vi "Example Three Stage.vi"() -> ()   [LabVIEW 2019]
uses:
  Class/Controller/Controller.lvclass
  <vilib>/Platform/TimedLoop/XDataNode/timing_clust.ctl
  <vilib>/Platform/TimedLoop/XDataNode/nitl_modes.ctl
  <vilib>/Platform/TimedLoop/XDataNode/wakeup.ctl
  <vilib>/platform/TimedLoop/XDataNode/XDataNode.xnode
  <vilib>/Platform/TimedLoop/XDataNode/XDNodeRunTimeDep.lvlib
panel:
  in  "Tab Control 3":enum32{"Motion", "Settings"}(tab)
  in  "Zero Output 3":bool
  in  "Go to Home 3":bool
  in  "Scan Right 3":bool
  in  "Scan Left 3":bool
  in  "Continue 3":bool
  in  "Stop 3":bool
  in  "Make Step Right 3":bool
  in  "Step Size \n[selected units] 3":dbl=1.0 format="%#.2f"
  in  "Make Step Left 3":bool
  in  "Desired Speed \n[1µm/s or 0,01deg /s] 3":dbl=10000.0 format="%#.2f"
  in  "Desired Position \n[selected units] 3":dbl format="%#.2f"
  in  "Find Index 3":bool
  in  "Reset 3":bool
  out "Desired Position\n[selected units] 3":dbl
  out "Encoder position \n[selected units] 3":dbl
  out "Waveform Chart 3":dbl(graph)=-0.078
  out "Status Info 3":T1
  out "StatusBits 3":T2
  in  "Working Units 3":string(combo)="1000000"
  in  "Axis Resolution 3":string(combo)="312,5"
  in  "Axis Letter 3":string="Z"
  in  "Tab Control 2":enum32{"Motion", "Settings"}(tab)
  in  "Zero Output 2":bool
  in  "Go to Home 2":bool
  in  "Scan Right 2":bool
  in  "Scan Left 2":bool
  in  "Continue 2":bool
  in  "Stop 2":bool
  in  "Make Step Right 2":bool
  in  "Step Size \n[selected units] 2":dbl=1.0 format="%#.2f"
  in  "Make Step Left 2":bool
  in  "Desired Speed \n[1µm/s or 0,01deg /s] 2":dbl=10000.0 format="%#.2f"
  in  "Desired Position \n[selected units] 2":dbl format="%#.2f"
  in  "Find Index 2":bool
  in  "Reset 2":bool
  out "Desired Position\n[selected units] 2":dbl
  out "Encoder position \n[selected units] 2":dbl
  out "Waveform Chart 2":dbl(graph)=-0.078
  out "Status Info 2":T1
  out "StatusBits 2":T2
  out "Desired Position\n[selected units]":dbl
  out "Encoder position \n[selected units]":dbl
  in  "Tab Control":enum32{"Motion", "Settings"}(tab)
  in  "Zero Output":bool
  in  "Go to Home":bool
  in  "Scan Right":bool
  in  "Scan Left":bool
  in  "Continue":bool
  in  "Stop":bool
  in  "Make Step Right":bool
  in  "Step Size \n[selected units]":dbl=1.0 format="%#.2f"
  in  "Make Step Left":bool
  in  "Desired Speed \n[1µm/s or 0,01deg /s]":dbl=10000.0 format="%#.2f"
  in  "Desired Position \n[selected units]":dbl format="%#.2f"
  in  "Find Index":bool
  in  "Reset":bool
  out "error out":errorcluster
  in  "Working Units 2":string(combo)="1000000"
  in  "Working Units":string(combo)="1000000"
  out "StatusBits":T2
  out "Status Info":T1
  in  "Axis Resolution 2":string(combo)="312,5"
  in  "Axis Letter 2":string="Y"
  in  "Axis Resolution":string(combo)="312,5"
  in  "Axis Letter":string="X"
  in  "Baudrate":dbl=9600.0
  in  "COM Port":refnum<visa-resource-name>
  in  "Controller.lvclass":refnum<class "Controller.lvclass">
  out "Waveform Chart":dbl(graph)=-0.078
  in  "STOP PROGRAM":bool
  # "Visualization"
  # "Extra information"
  # "READ ME FIRST"
  # "Configuration"
  # "Stage 1"
  # "Driver 1"
  # "Stage 1"
  # "How to run:"
  # "BEFORE RUNNING:"
  # "1, Select COM Port"
  # "2. Select baudrate"
  # "3. For each axis:"
  # "3.1 Specify correct axis name (1 letter)"
  # "3.2 Specify correct resolution"
  # "4. Run VI"
  # "WHEN RUNNING, YOU HAVE TO FIRST PUSH \"FIND INDEX\" FOR EACH STAGE.\nThe stages will start moving and find its position. After that you can control the stages"
  # "Stage 2"
  # "NOTES: Do this only the first time"
  # "1. Replace the settings_default.txt file with\nthe file we provided on a USB stick."
  # "2.    Make sure there are no comments in the\nsettings_default.txt file. ONLY lines like: \"X:DPOS=100\" so NO \"%\" in front or at the end of the line."
  # "Position Information"
  # "Stage 3"
  # "3.  In your settings_default.txt file:\nEvery line that contains SSPD or MSPD: multiply that value with:\n - 1000 for a lineair stage \n - 100 for a rotating stage"
  # "STOP BUTTON"
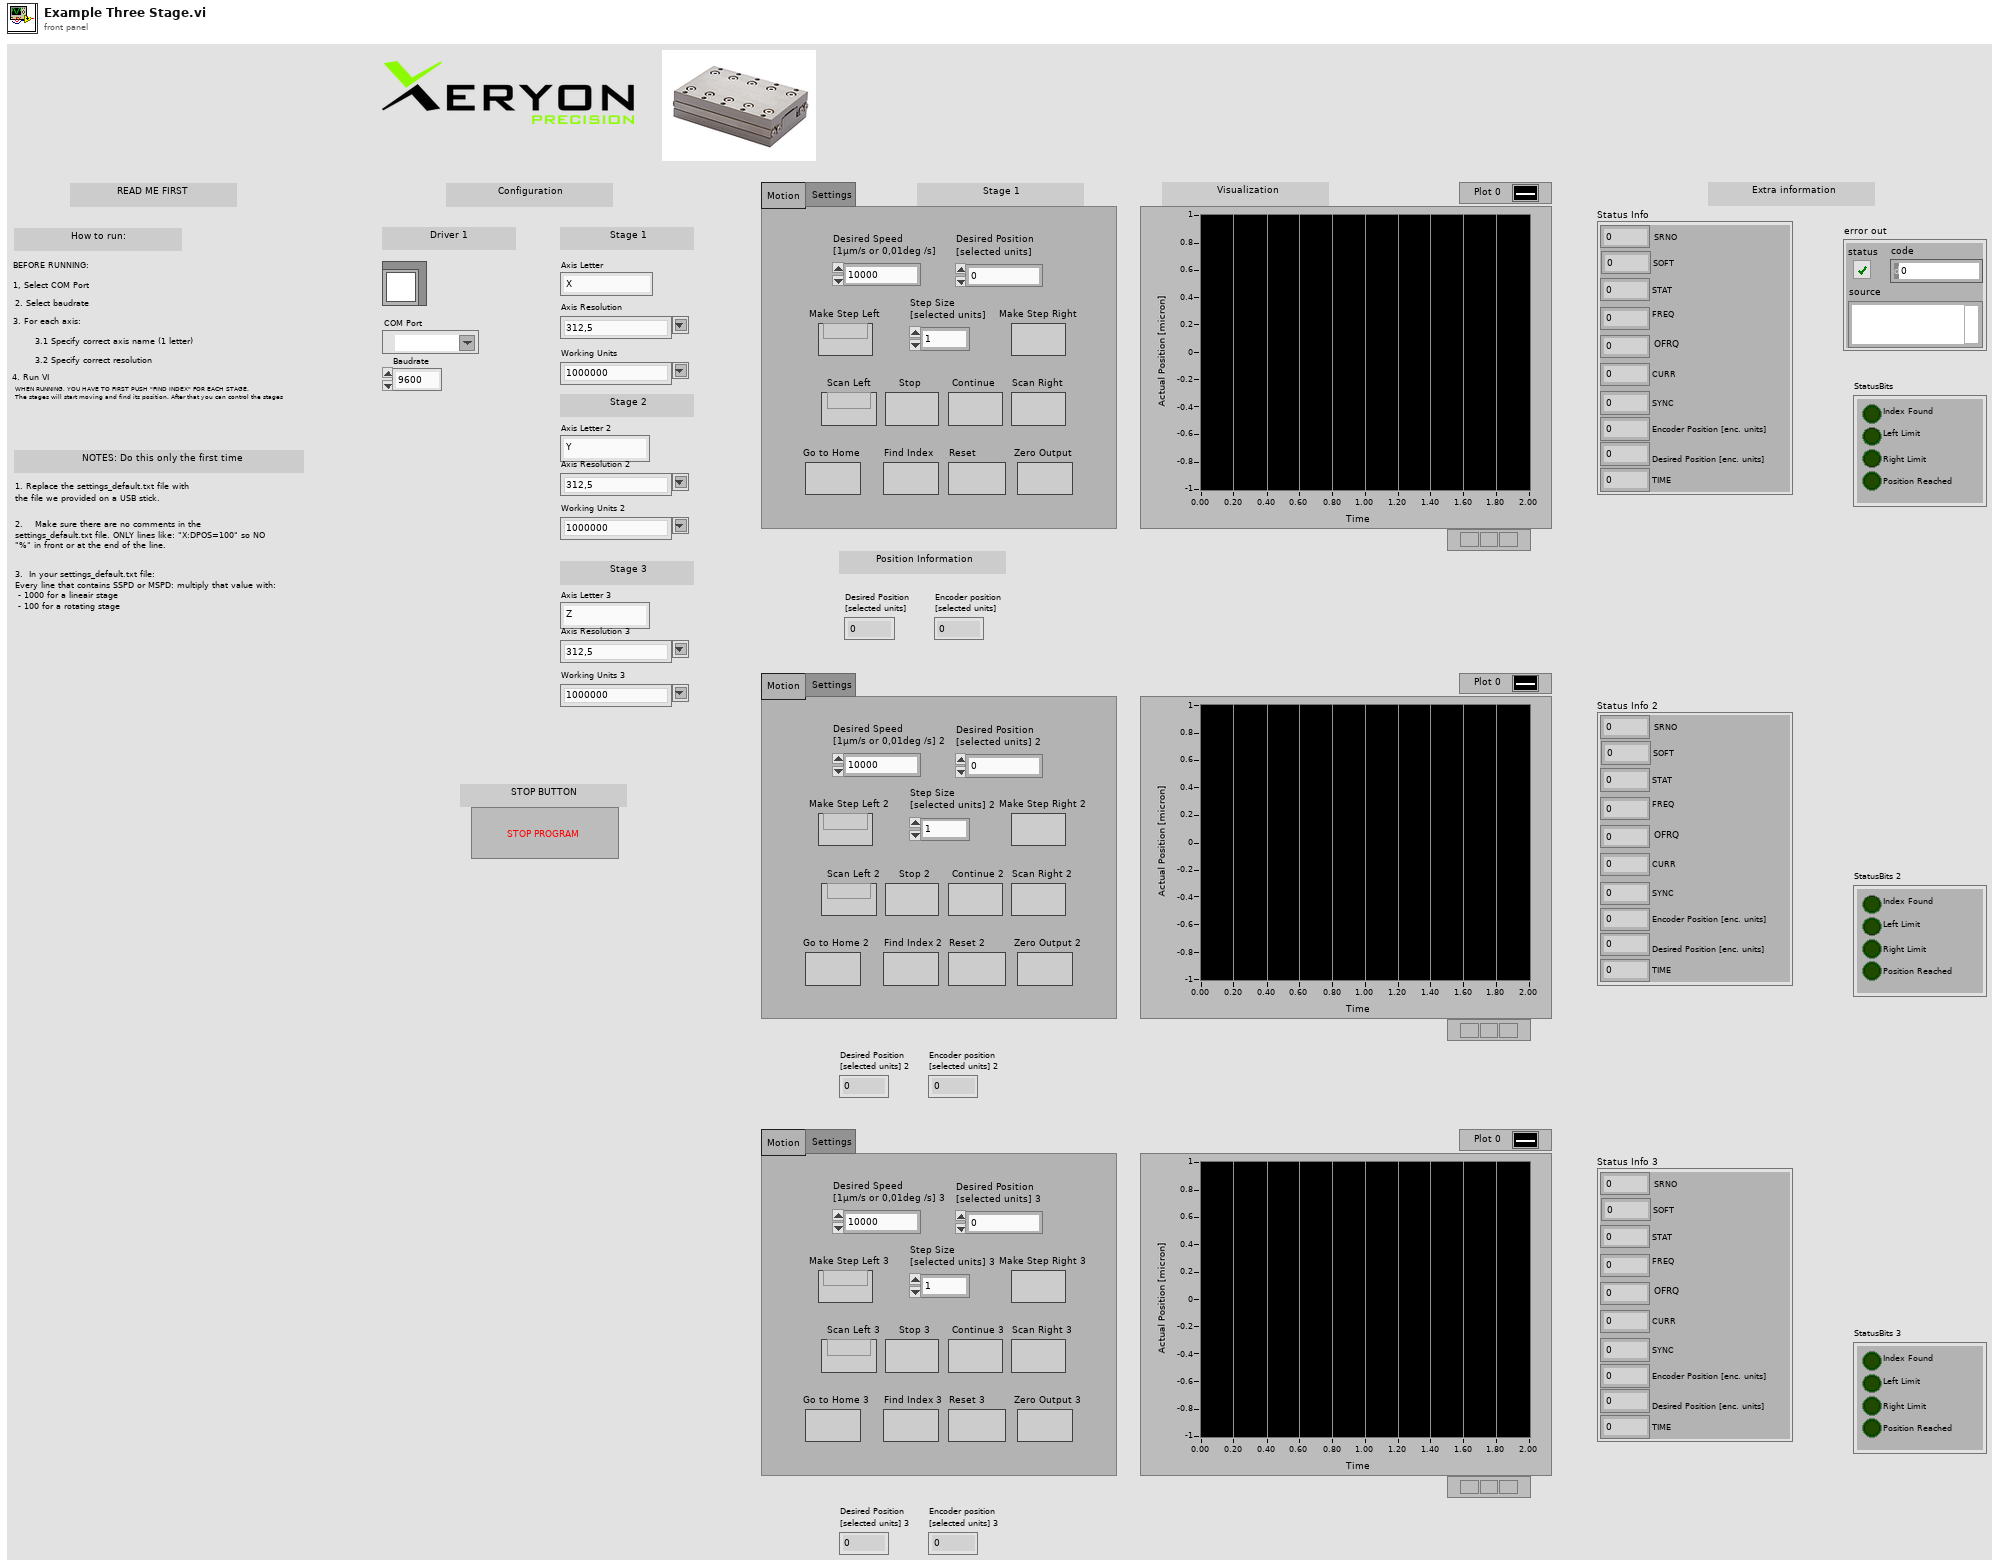
[diagram p1: front panel]
types:
  T1 = cluster{"SRNO":dbl, "SOFT":dbl, "STAT":dbl, "FREQ":dbl, "OFRQ":dbl, "CURR":dbl, "SYNC":dbl, "Encoder Position [enc. units]":dbl, "Desired Position [enc. units]":dbl, "TIME":dbl}
  T2 = cluster{"Index Found":bool, "Left Limit":bool, "Right Limit":bool, "Position Reached":bool}
  T3 = typedef "XDNodeRunTimeDep.lvlib/timing_clust.ctl" = cluster{"Expected End [f-1]":u64, "Actual End [f-1]":u64, "Finished Late? [f-1]":bool, "Expected End [i-1]":u64, "Actual End [i-1]":u64, "Finished Late? [i-1]":bool, "Expected Start [i]":u64, "Actual Start [i]":u64, "Expected Start [f]":u64, "Actual Start [f]":u64, "Source Name":string, "Structure Name":string, "Period":i64, "Deadline":i64, "Offset":i64, "Start":i64, "Priority":i32, "Timeout":i32, "Mode":T4, "Wakeup Reason":T5, "Error":errorcluster, "Source Type":string, "Secondary Source Type":string, "Global End Time":u64, "Global Start Time":u64, "Frame Duration":u64, "Iteration Duration":u64, "Assigned CPU":i32, "I/O Scan Engine Mode":u32}
  T4 = typedef "XDNodeRunTimeDep.lvlib/nitl_modes.ctl" = enum32{"No Change", "Process missed periods, maintain original phase", "Discard missed periods, maintain original phase", "Process missed periods, ignore original phase", "Discard missed periods, ignore original phase"}
  T5 = typedef "XDNodeRunTimeDep.lvlib/wakeup.ctl" = enum32{"Normal", "Aborted", "Asynchronous wakeup", "Timing source error", "Timed loop error", "Timeout"}
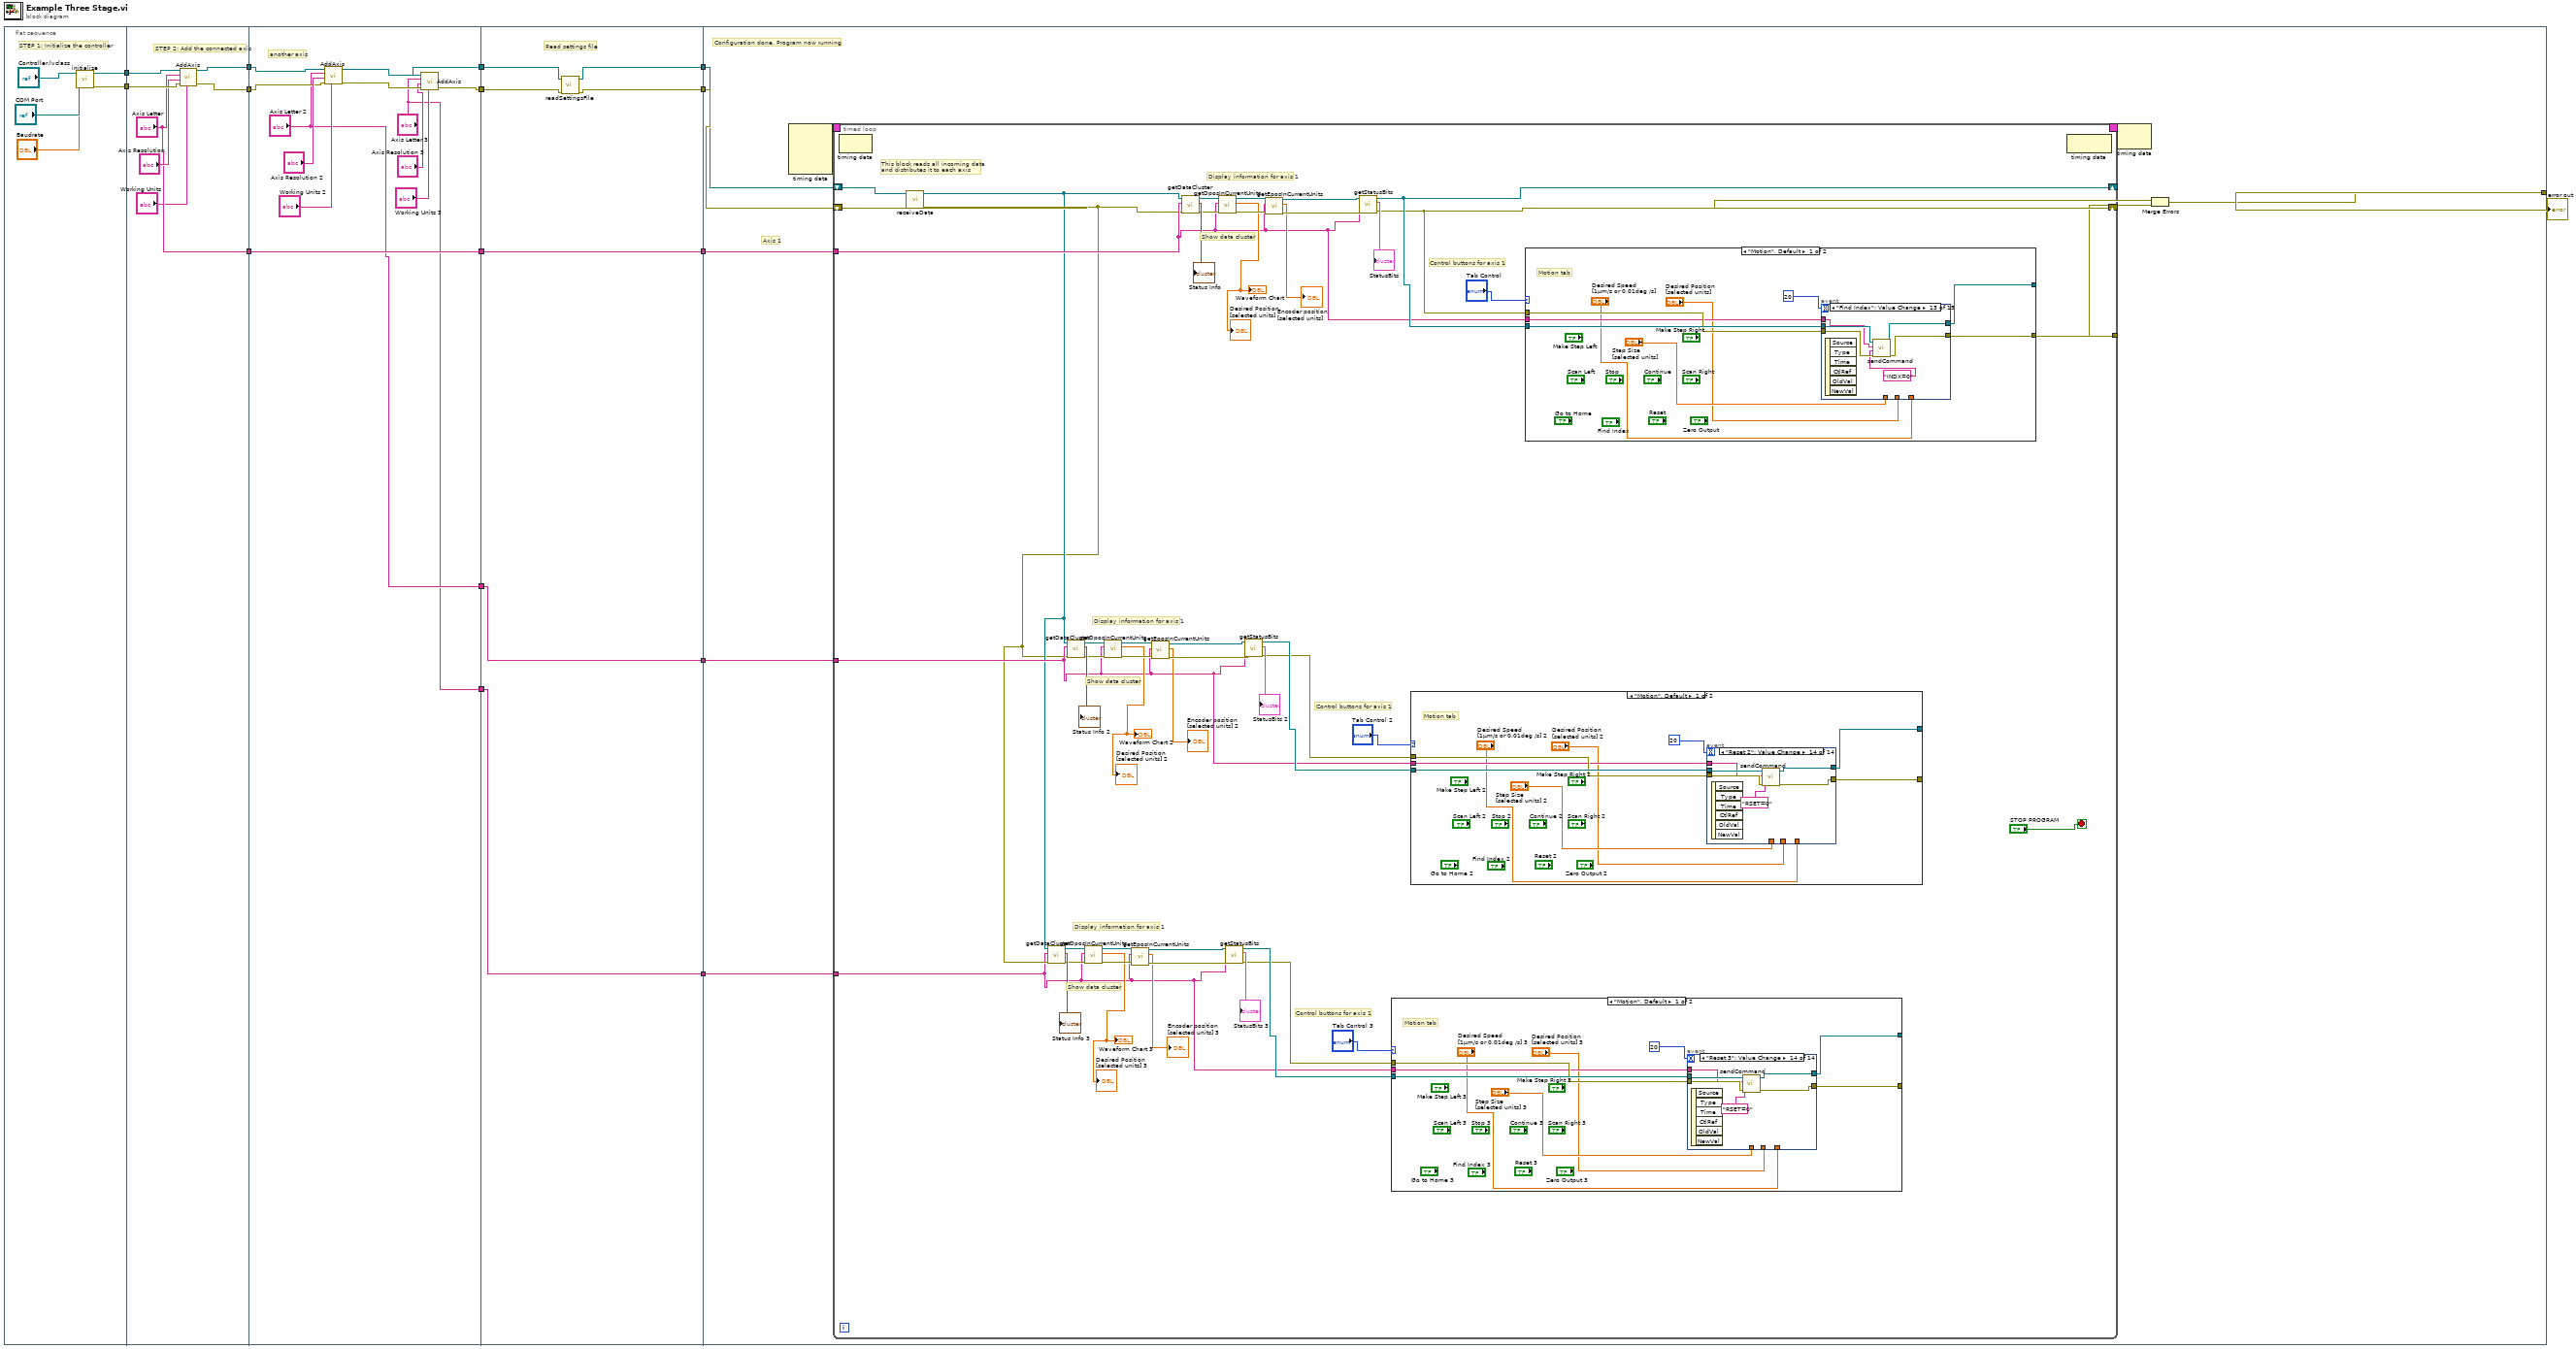
[diagram p0: block diagram]
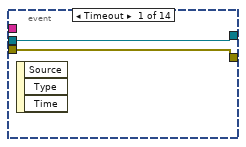
[diagram p2: hidden frame]
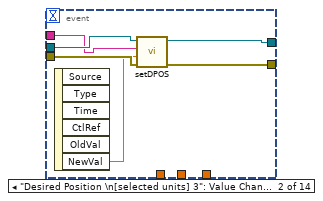
[diagram p3: hidden frame]
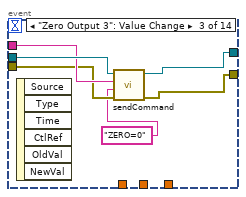
[diagram p4: hidden frame]
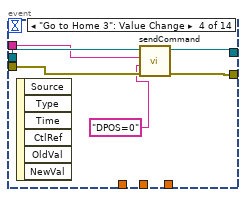
[diagram p5: hidden frame]
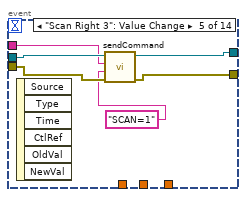
[diagram p6: hidden frame]
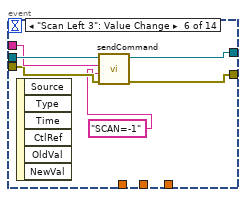
[diagram p7: hidden frame]
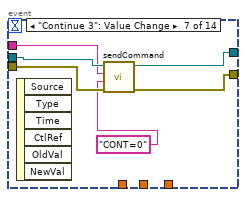
[diagram p8: hidden frame]
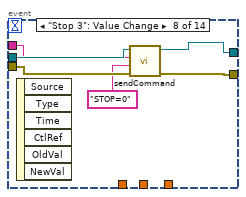
[diagram p9: hidden frame]
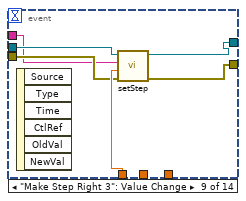
[diagram p10: hidden frame]
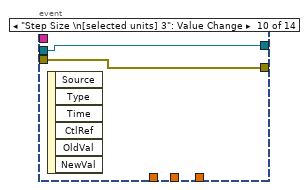
[diagram p11: hidden frame]
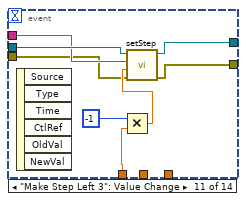
[diagram p12: hidden frame]
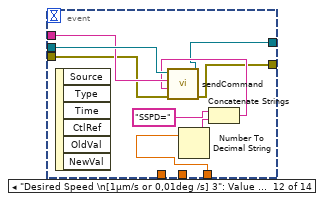
[diagram p13: hidden frame]
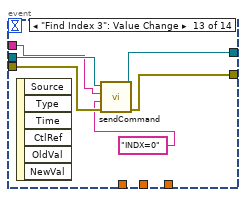
[diagram p14: hidden frame]
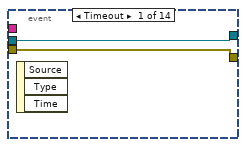
[diagram p16: hidden frame]
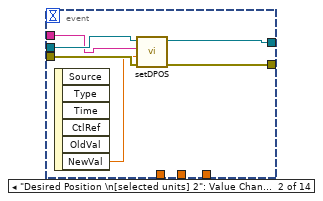
[diagram p17: hidden frame]
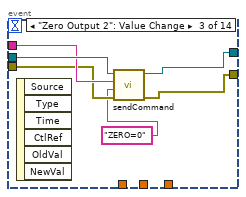
[diagram p18: hidden frame]
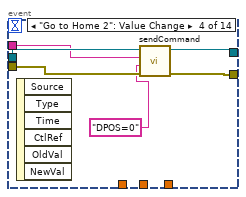
[diagram p19: hidden frame]
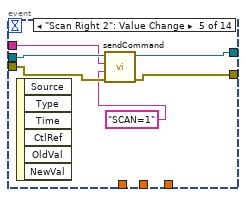
[diagram p20: hidden frame]
diagram:
  n1 = flat-sequence {
    tunnel: [w18] -> w16
    tunnel: [w17] -> w15
    tunnel: w16 -> [w28]
    tunnel: w15 -> [w27]
    tunnel: [w25] -> w14
    tunnel: [w24] -> w13
    tunnel: ["Axis Letter"] -> w12
    tunnel: w14 -> [w39]
    tunnel: w13 -> [w38]
    tunnel: [w41] -> w10
    tunnel: w12 -> [w41]
    tunnel: [w34] -> w8
    tunnel: [w32] -> w6
    tunnel: ["Axis Letter 2"] -> w4
    tunnel: ["Axis Letter 3"] -> w1
    tunnel: w10 -> [w48]
    tunnel: [w48] -> w9
    tunnel: w8 -> [w47]
    tunnel: [w45] -> w7
    tunnel: w6 -> [w46]
    tunnel: [w44] -> w5
    tunnel: w4 -> [w43]
    tunnel: [w43] -> w3
    tunnel: [w42] -> w2
    tunnel: w1 -> [w42]
    tunnel: w9 -> [w51]
    tunnel: w7 -> [w57]
    tunnel: w5 -> [w58]
    tunnel: [w53] -> w11
    tunnel: w3 -> [w50]
    tunnel: w2 -> [w49]
    frame #0 {
      # "STEP 1: Initialize the controller"
      n2 = call-dynamic "initialize.vi"("Baudrate"="Baudrate", "COM Port"="COM Port", "Controller in"="Controller.lvclass") -> ("error out"=w17:errorcluster, "Controller out"=w18:refnum<class "Controller.lvclass">)  [unwired: 7 in]
    }
    frame #1 {
      # "STEP 2: Add the connected axis"
      n3 = call-dynamic "AddAxis.vi"("Units"="Working Units", "error in (no error)"=w27, "Encoder Resolution"="Axis Resolution", "Axis Letter"="Axis Letter", "Controller in"=w28) -> ("error out"=w24:errorcluster, "Controller out"=w25:refnum<class "Controller.lvclass">)  [unwired: 5 in]
    }
    frame #2 {
      # "another axis"
      n4 = call-dynamic "AddAxis.vi"("Units"="Working Units 2", "error in (no error)"=w38, "Encoder Resolution"="Axis Resolution 2", "Axis Letter"="Axis Letter 2", "Controller in"=w39) -> ("error out"=w33:errorcluster, "Controller out"=w35:refnum<class "Controller.lvclass">)  [unwired: 5 in]
      n5 = call-dynamic "AddAxis.vi"("Units"="Working Units 3", "error in (no error)"=w33, "Encoder Resolution"="Axis Resolution 3", "Axis Letter"="Axis Letter 3", "Controller in"=w35) -> ("error out"=w32:errorcluster, "Controller out"=w34:refnum<class "Controller.lvclass">)  [unwired: 5 in]
    }
    frame #3 {
      # "Read settings file"
      n6 = call-dynamic "readSettingsFile.vi"("error in (no error)"=w46, "Controller in"=w47) -> ("error out"=w44:errorcluster, "Controller out"=w45:refnum<class "Controller.lvclass">)  [unwired: 8 in]
    }
    frame #4 {
      # "Axis 1"
      # "Configuration done. Program now running"
      n7 = node-c288() -> (w56:T3)  [unwired: 4 in]
      n8 = timed-loop {
        shift-right: [w92] -> _
        shift-left: w57 -> [w106]
        tunnel: w51 -> [w90]
        shift-right: [w91] -> w54
        shift-left: w58 -> [w95]
        timing: w56 -> [_]
        timing-out: [_] -> w55
        tunnel: [w89] -> w52
        tunnel: w50 -> [w75]
        tunnel: w49 -> [w59]
        stop <- "STOP PROGRAM" stop-if-true
        # "Control buttons for axis 1"
        # "Display information for axis 1"
        # "Show data cluster"
        # "Control buttons for axis 1"
        # "Display information for axis 1"
        # "Show data cluster"
        # "Control buttons for axis 1"
        # "Display information for axis 1"
        # "Show data cluster"
        # "This block reads all incoming data\nand distributes it to each axis"
        n9 = node-c288() -> ()  [unwired: 1 in, 1 out]
        n10 = call-dynamic "receiveData.vi"("error in (no error)"=w95, "Controller in"=w106) -> ("error out"=w60:errorcluster, "Controller out"=w61:refnum<class "Controller.lvclass">)  [unwired: 8 in]
        n11 = call-dynamic "getDataCluster.vi"("error in (no error)"=w60, "Axis Letter"=w59, "Controller in"=w61) -> ("error out"=w69:errorcluster, "Information"=→"Status Info 3":T1, "Controller out"=w72:refnum<class "Controller.lvclass">)  [unwired: 6 in]
        n12 = call-dynamic "getDataCluster.vi"("error in (no error)"=w60, "Axis Letter"=w75, "Controller in"=w61) -> ("error out"=w83:errorcluster, "Information"=→"Status Info 2":T1, "Controller out"=w86:refnum<class "Controller.lvclass">)  [unwired: 6 in]
        n13 = call-dynamic "getDposInCurrentUnits.vi"("error in (no error)"=w69, "Axis Letter"=w59, "Controller in"=w72) -> ("error out"=w68:errorcluster, "DPOS In Current Units"=→"Waveform Chart 3" →"Desired Position\n[selected units] 3":dbl, "Controller out"=w71:refnum<class "Controller.lvclass">)  [unwired: 6 in]
        n14 = call-dynamic "getDposInCurrentUnits.vi"("error in (no error)"=w83, "Axis Letter"=w75, "Controller in"=w86) -> ("error out"=w82:errorcluster, "DPOS In Current Units"=→"Waveform Chart 2" →"Desired Position\n[selected units] 2":dbl, "Controller out"=w85:refnum<class "Controller.lvclass">)  [unwired: 6 in]
        n15 = call-dynamic "getEposInCurrentUnits.vi"("error in (no error)"=w68, "Axis Letter"=w59, "Controller in"=w71) -> ("error out"=w67:errorcluster, "EPOS In Current Units"=→"Encoder position \n[selected units] 3":dbl, "Controller out"=w70:refnum<class "Controller.lvclass">)  [unwired: 6 in]
        n16 = call-dynamic "getEposInCurrentUnits.vi"("error in (no error)"=w82, "Axis Letter"=w75, "Controller in"=w85) -> ("error out"=w81:errorcluster, "EPOS In Current Units"=→"Encoder position \n[selected units] 2":dbl, "Controller out"=w84:refnum<class "Controller.lvclass">)  [unwired: 6 in]
        n17 = call-dynamic "getDataCluster.vi"("error in (no error)"=w60, "Axis Letter"=w90, "Controller in"=w61) -> ("error out"=w100:errorcluster, "Information"=→"Status Info":T1, "Controller out"=w103:refnum<class "Controller.lvclass">)  [unwired: 6 in]
        n18 = call-dynamic "getDposInCurrentUnits.vi"("error in (no error)"=w100, "Axis Letter"=w90, "Controller in"=w103) -> ("error out"=w99:errorcluster, "DPOS In Current Units"=→"Waveform Chart" →"Desired Position\n[selected units]":dbl, "Controller out"=w102:refnum<class "Controller.lvclass">)  [unwired: 6 in]
        n19 = call-dynamic "getStatusBits.vi"("error in (no error)"=w67, "Axis Letter"=w59, "Controller in"=w70) -> ("error out"=w62:errorcluster, "StatusBits"=→"StatusBits 3":T2, "Controller out"=w63:refnum<class "Controller.lvclass">)  [unwired: 6 in]
        n20 = call-dynamic "getStatusBits.vi"("error in (no error)"=w81, "Axis Letter"=w75, "Controller in"=w84) -> ("error out"=w76:errorcluster, "StatusBits"=→"StatusBits 2":T2, "Controller out"=w77:refnum<class "Controller.lvclass">)  [unwired: 6 in]
        n21 = call-dynamic "getEposInCurrentUnits.vi"("error in (no error)"=w99, "Axis Letter"=w90, "Controller in"=w102) -> ("error out"=w98:errorcluster, "EPOS In Current Units"=→"Encoder position \n[selected units]":dbl, "Controller out"=w101:refnum<class "Controller.lvclass">)  [unwired: 6 in]
        n22 = call-dynamic "getStatusBits.vi"("error in (no error)"=w98, "Axis Letter"=w90, "Controller in"=w101) -> ("error out"=w91:errorcluster, "StatusBits"=→"StatusBits":T2, "Controller out"=w92:refnum<class "Controller.lvclass">)  [unwired: 6 in]
        n23 = case shown="\"Motion\", Default" "Tab Control 3" {
          tunnel: w63 -> [w115 w197]
          tunnel: w62 -> [w114 w198]
          tunnel: [w113 w197] -> _
          tunnel: [w112 w198] -> _
          tunnel: w59 -> [w110 _]
          frame "Motion", Default {
            # "Motion tab"
            n24 = event shown="[13] \"Reset 3\": Value Change" {
              selector: _ -> [_ _ _ _ _ _ _ _ _ _ _ _ _ _]
              dyn-events: _ -> [_ _ _ _ _ _ _ _ _ _ _ _ _ _]
              timeout: 20 -> [_ _ _ _ _ _ _ _ _ _ _ _ _ _]
              tunnel: w115 -> [w117 w123 w129 w135 w141 w147 w153 w159 w163 w167 w173 w184 w190 w196]
              tunnel: w114 -> [w116 w122 w127 w133 w139 w145 w151 w157 w164 w166 w170 w182 w188 w195]
              tunnel: [w117 w120 w125 w130 w137 w143 w149 w155 w161 w167 w168 w176 w186 w192] -> w113
              tunnel: [w116 w121 w126 w132 w138 w144 w150 w156 w160 w166 w169 w177 w187 w191] -> w112
              tunnel: w110 -> [_ w118 w128 w134 w140 w146 w152 w158 w162 _ w172 w183 w189 w194]
              tunnel: "Step Size \n[selected units] 3" -> [_ _ _ _ _ _ _ _ w165 _ w174 _ _ _]
              tunnel: "Desired Position \n[selected units] 3" -> [_ _ _ _ _ _ _ _ _ _ _ _ _ _]
              tunnel: "Desired Speed \n[1µm/s or 0,01deg /s] 3" -> [_ _ _ _ _ _ _ _ _ _ _ w181 _ _]
              event Timeout {
                n25 = event-data() -> ()  [unwired: 1 in, 3 out]
              }
              event "Desired Position \n[selected units] 3": Value Change {
                n26 = event-data() -> ("NewVal"=w119:dbl)  [unwired: 1 in, 5 out]
                n27 = call-dynamic "setDPOS.vi"("error in (no error)"=w122, "DPOS In Current Units"=w119, "Axis Letter"=w118, "Controller in"=w123) -> ("error out"=w121:errorcluster, "Controller out"=w120:refnum<class "Controller.lvclass">)  [unwired: 6 in]
              }
              event "Zero Output 3": Value Change {
                n28 = event-data() -> ()  [unwired: 1 in, 6 out]
                n29 = call-dynamic "sendCommand.vi"("error in (no error)"=w127, "Command"="ZERO=0", "Axis Letter"=w128, "Controller in"=w129) -> ("error out"=w126:errorcluster, "Controller out"=w125:refnum<class "Controller.lvclass">)  [unwired: 6 in]
              }
              event "Go to Home 3": Value Change {
                n30 = event-data() -> ()  [unwired: 1 in, 6 out]
                n31 = call-dynamic "sendCommand.vi"("error in (no error)"=w133, "Command"="DPOS=0", "Axis Letter"=w134, "Controller in"=w135) -> ("error out"=w132:errorcluster, "Controller out"=w130:refnum<class "Controller.lvclass">)  [unwired: 6 in]
              }
              event "Scan Right 3": Value Change {
                n32 = event-data() -> ()  [unwired: 1 in, 6 out]
                n33 = call-dynamic "sendCommand.vi"("error in (no error)"=w139, "Command"="SCAN=1", "Axis Letter"=w140, "Controller in"=w141) -> ("error out"=w138:errorcluster, "Controller out"=w137:refnum<class "Controller.lvclass">)  [unwired: 6 in]
              }
              event "Scan Left 3": Value Change {
                n34 = event-data() -> ()  [unwired: 1 in, 6 out]
                n35 = call-dynamic "sendCommand.vi"("error in (no error)"=w145, "Command"="SCAN=-1", "Axis Letter"=w146, "Controller in"=w147) -> ("error out"=w144:errorcluster, "Controller out"=w143:refnum<class "Controller.lvclass">)  [unwired: 6 in]
              }
              event "Continue 3": Value Change {
                n36 = event-data() -> ()  [unwired: 1 in, 6 out]
                n37 = call-dynamic "sendCommand.vi"("error in (no error)"=w151, "Command"="CONT=0", "Axis Letter"=w152, "Controller in"=w153) -> ("error out"=w150:errorcluster, "Controller out"=w149:refnum<class "Controller.lvclass">)  [unwired: 6 in]
              }
              event "Stop 3": Value Change {
                n38 = event-data() -> ()  [unwired: 1 in, 6 out]
                n39 = call-dynamic "sendCommand.vi"("error in (no error)"=w157, "Command"="STOP=0", "Axis Letter"=w158, "Controller in"=w159) -> ("error out"=w156:errorcluster, "Controller out"=w155:refnum<class "Controller.lvclass">)  [unwired: 6 in]
              }
              event "Make Step Right 3": Value Change {
                n40 = event-data() -> ()  [unwired: 1 in, 6 out]
                n41 = call-dynamic "setStep.vi"("error in (no error)"=w164, "Step Value"=w165, "Axis Letter"=w162, "Controller in"=w163) -> ("error out"=w160:errorcluster, "Controller out"=w161:refnum<class "Controller.lvclass">)  [unwired: 6 in]
              }
              event "Step Size \n[selected units] 3": Value Change {
                n42 = event-data() -> ()  [unwired: 1 in, 6 out]
              }
              event "Make Step Left 3": Value Change {
                n43 = event-data() -> ()  [unwired: 1 in, 6 out]
                n44 = Multiply(x=-1, y=w174) -> (x*y=w171:dbl)
                n45 = call-dynamic "setStep.vi"("error in (no error)"=w170, "Step Value"=w171, "Axis Letter"=w172, "Controller in"=w173) -> ("error out"=w169:errorcluster, "Controller out"=w168:refnum<class "Controller.lvclass">)  [unwired: 6 in]
              }
              event "Desired Speed \n[1µm/s or 0,01deg /s] 3": Value Change {
                n46 = event-data() -> ()  [unwired: 1 in, 6 out]
                n47 = Number To Decimal String(number=w181) -> (decimal integer string=w179:string)  [unwired: 1 in]
                n48 = Concatenate Strings("SSPD=", w179) -> (w178:string)
                n49 = call-dynamic "sendCommand.vi"("error in (no error)"=w182, "Command"=w178, "Axis Letter"=w183, "Controller in"=w184) -> ("error out"=w177:errorcluster, "Controller out"=w176:refnum<class "Controller.lvclass">)  [unwired: 6 in]
              }
              event "Find Index 3": Value Change {
                n50 = event-data() -> ()  [unwired: 1 in, 6 out]
                n51 = call-dynamic "sendCommand.vi"("error in (no error)"=w188, "Command"="INDX=0", "Axis Letter"=w189, "Controller in"=w190) -> ("error out"=w187:errorcluster, "Controller out"=w186:refnum<class "Controller.lvclass">)  [unwired: 6 in]
              }
              event "Reset 3": Value Change {
                n52 = event-data() -> ()  [unwired: 1 in, 6 out]
                n53 = call-dynamic "sendCommand.vi"("error in (no error)"=w195, "Command"="RSET=0", "Axis Letter"=w194, "Controller in"=w196) -> ("error out"=w191:errorcluster, "Controller out"=w192:refnum<class "Controller.lvclass">)  [unwired: 6 in]
              }
            }
          }
          frame "Settings" {
          }
        }
        n54 = case shown="\"Motion\", Default" "Tab Control 2" {
          tunnel: w77 -> [w207 w289]
          tunnel: w76 -> [w206 w290]
          tunnel: [w205 w289] -> _
          tunnel: [w204 w290] -> _
          tunnel: w75 -> [w202 _]
          frame "Motion", Default {
            # "Motion tab"
            n55 = event shown="[13] \"Reset 2\": Value Change" {
              selector: _ -> [_ _ _ _ _ _ _ _ _ _ _ _ _ _]
              dyn-events: _ -> [_ _ _ _ _ _ _ _ _ _ _ _ _ _]
              timeout: 20 -> [_ _ _ _ _ _ _ _ _ _ _ _ _ _]
              tunnel: w207 -> [w209 w215 w221 w227 w233 w239 w245 w251 w255 w259 w265 w276 w282 w288]
              tunnel: w206 -> [w208 w214 w219 w225 w231 w237 w243 w249 w256 w258 w262 w274 w280 w287]
              tunnel: [w209 w212 w217 w222 w229 w235 w241 w247 w253 w259 w260 w268 w278 w284] -> w205
              tunnel: [w208 w213 w218 w224 w230 w236 w242 w248 w252 w258 w261 w269 w279 w283] -> w204
              tunnel: w202 -> [_ w210 w220 w226 w232 w238 w244 w250 w254 _ w264 w275 w281 w286]
              tunnel: "Step Size \n[selected units] 2" -> [_ _ _ _ _ _ _ _ w257 _ w266 _ _ _]
              tunnel: "Desired Position \n[selected units] 2" -> [_ _ _ _ _ _ _ _ _ _ _ _ _ _]
              tunnel: "Desired Speed \n[1µm/s or 0,01deg /s] 2" -> [_ _ _ _ _ _ _ _ _ _ _ w273 _ _]
              event Timeout {
                n56 = event-data() -> ()  [unwired: 1 in, 3 out]
              }
              event "Desired Position \n[selected units] 2": Value Change {
                n57 = event-data() -> ("NewVal"=w211:dbl)  [unwired: 1 in, 5 out]
                n58 = call-dynamic "setDPOS.vi"("error in (no error)"=w214, "DPOS In Current Units"=w211, "Axis Letter"=w210, "Controller in"=w215) -> ("error out"=w213:errorcluster, "Controller out"=w212:refnum<class "Controller.lvclass">)  [unwired: 6 in]
              }
              event "Zero Output 2": Value Change {
                n59 = event-data() -> ()  [unwired: 1 in, 6 out]
                n60 = call-dynamic "sendCommand.vi"("error in (no error)"=w219, "Command"="ZERO=0", "Axis Letter"=w220, "Controller in"=w221) -> ("error out"=w218:errorcluster, "Controller out"=w217:refnum<class "Controller.lvclass">)  [unwired: 6 in]
              }
              event "Go to Home 2": Value Change {
                n61 = event-data() -> ()  [unwired: 1 in, 6 out]
                n62 = call-dynamic "sendCommand.vi"("error in (no error)"=w225, "Command"="DPOS=0", "Axis Letter"=w226, "Controller in"=w227) -> ("error out"=w224:errorcluster, "Controller out"=w222:refnum<class "Controller.lvclass">)  [unwired: 6 in]
              }
              event "Scan Right 2": Value Change {
                n63 = event-data() -> ()  [unwired: 1 in, 6 out]
                n64 = call-dynamic "sendCommand.vi"("error in (no error)"=w231, "Command"="SCAN=1", "Axis Letter"=w232, "Controller in"=w233) -> ("error out"=w230:errorcluster, "Controller out"=w229:refnum<class "Controller.lvclass">)  [unwired: 6 in]
              }
              event "Scan Left 2": Value Change {
                n65 = event-data() -> ()  [unwired: 1 in, 6 out]
                n66 = call-dynamic "sendCommand.vi"("error in (no error)"=w237, "Command"="SCAN=-1", "Axis Letter"=w238, "Controller in"=w239) -> ("error out"=w236:errorcluster, "Controller out"=w235:refnum<class "Controller.lvclass">)  [unwired: 6 in]
              }
              event "Continue 2": Value Change {
                n67 = event-data() -> ()  [unwired: 1 in, 6 out]
                n68 = call-dynamic "sendCommand.vi"("error in (no error)"=w243, "Command"="CONT=0", "Axis Letter"=w244, "Controller in"=w245) -> ("error out"=w242:errorcluster, "Controller out"=w241:refnum<class "Controller.lvclass">)  [unwired: 6 in]
              }
              event "Stop 2": Value Change {
                n69 = event-data() -> ()  [unwired: 1 in, 6 out]
                n70 = call-dynamic "sendCommand.vi"("error in (no error)"=w249, "Command"="STOP=0", "Axis Letter"=w250, "Controller in"=w251) -> ("error out"=w248:errorcluster, "Controller out"=w247:refnum<class "Controller.lvclass">)  [unwired: 6 in]
              }
              event "Make Step Right 2": Value Change {
                n71 = event-data() -> ()  [unwired: 1 in, 6 out]
                n72 = call-dynamic "setStep.vi"("error in (no error)"=w256, "Step Value"=w257, "Axis Letter"=w254, "Controller in"=w255) -> ("error out"=w252:errorcluster, "Controller out"=w253:refnum<class "Controller.lvclass">)  [unwired: 6 in]
              }
              event "Step Size \n[selected units] 2": Value Change {
                n73 = event-data() -> ()  [unwired: 1 in, 6 out]
              }
              event "Make Step Left 2": Value Change {
                n74 = event-data() -> ()  [unwired: 1 in, 6 out]
                n75 = Multiply(x=-1, y=w266) -> (x*y=w263:dbl)
                n76 = call-dynamic "setStep.vi"("error in (no error)"=w262, "Step Value"=w263, "Axis Letter"=w264, "Controller in"=w265) -> ("error out"=w261:errorcluster, "Controller out"=w260:refnum<class "Controller.lvclass">)  [unwired: 6 in]
              }
              event "Desired Speed \n[1µm/s or 0,01deg /s] 2": Value Change {
                n77 = event-data() -> ()  [unwired: 1 in, 6 out]
                n78 = Number To Decimal String(number=w273) -> (decimal integer string=w271:string)  [unwired: 1 in]
                n79 = Concatenate Strings("SSPD=", w271) -> (w270:string)
                n80 = call-dynamic "sendCommand.vi"("error in (no error)"=w274, "Command"=w270, "Axis Letter"=w275, "Controller in"=w276) -> ("error out"=w269:errorcluster, "Controller out"=w268:refnum<class "Controller.lvclass">)  [unwired: 6 in]
              }
              event "Find Index 2": Value Change {
                n81 = event-data() -> ()  [unwired: 1 in, 6 out]
                n82 = call-dynamic "sendCommand.vi"("error in (no error)"=w280, "Command"="INDX=0", "Axis Letter"=w281, "Controller in"=w282) -> ("error out"=w279:errorcluster, "Controller out"=w278:refnum<class "Controller.lvclass">)  [unwired: 6 in]
              }
              event "Reset 2": Value Change {
                n83 = event-data() -> ()  [unwired: 1 in, 6 out]
                n84 = call-dynamic "sendCommand.vi"("error in (no error)"=w287, "Command"="RSET=0", "Axis Letter"=w286, "Controller in"=w288) -> ("error out"=w283:errorcluster, "Controller out"=w284:refnum<class "Controller.lvclass">)  [unwired: 6 in]
              }
            }
          }
          frame "Settings" {
          }
        }
        n85 = case shown="\"Motion\", Default" "Tab Control" {
          tunnel: w92 -> [w299 w381]
          tunnel: w91 -> [w298 w382]
          tunnel: [w297 w381] -> _
          tunnel: [w296 w382] -> w89
          tunnel: w90 -> [w294 _]
          frame "Motion", Default {
            # "Motion tab"
            n86 = event shown="[12] \"Find Index\": Value Change" {
              selector: _ -> [_ _ _ _ _ _ _ _ _ _ _ _ _ _ _]
              dyn-events: _ -> [_ _ _ _ _ _ _ _ _ _ _ _ _ _ _]
              timeout: 20 -> [_ _ _ _ _ _ _ _ _ _ _ _ _ _ _]
              tunnel: w299 -> [w301 w307 w313 w319 w325 w331 w337 w343 w347 w351 w357 w368 w374 w380 _]
              tunnel: w298 -> [w300 w306 w311 w317 w323 w329 w335 w341 w348 w350 w354 w366 w372 w379 _]
              tunnel: [w301 w304 w309 w314 w321 w327 w333 w339 w345 w351 w352 w360 w370 w376 _] -> w297
              tunnel: [w300 w305 w310 w316 w322 w328 w334 w340 w344 w350 w353 w361 w371 w375 _] -> w296
              tunnel: w294 -> [_ w302 w312 w318 w324 w330 w336 w342 w346 _ w356 w367 w373 w378 _]
              tunnel: "Step Size \n[selected units]" -> [_ _ _ _ _ _ _ _ w349 _ w358 _ _ _ _]
              tunnel: "Desired Position \n[selected units]" -> [_ _ _ _ _ _ _ _ _ _ _ _ _ _ _]
              tunnel: "Desired Speed \n[1µm/s or 0,01deg /s]" -> [_ _ _ _ _ _ _ _ _ _ _ w365 _ _ _]
              event Timeout {
                n87 = event-data() -> ()  [unwired: 1 in, 3 out]
              }
              event "Desired Position \n[selected units]": Value Change {
                n88 = event-data() -> ("NewVal"=w303:dbl)  [unwired: 1 in, 5 out]
                n89 = call-dynamic "setDPOS.vi"("error in (no error)"=w306, "DPOS In Current Units"=w303, "Axis Letter"=w302, "Controller in"=w307) -> ("error out"=w305:errorcluster, "Controller out"=w304:refnum<class "Controller.lvclass">)  [unwired: 6 in]
              }
              event "Zero Output": Value Change {
                n90 = event-data() -> ()  [unwired: 1 in, 6 out]
                n91 = call-dynamic "sendCommand.vi"("error in (no error)"=w311, "Command"="ZERO=0", "Axis Letter"=w312, "Controller in"=w313) -> ("error out"=w310:errorcluster, "Controller out"=w309:refnum<class "Controller.lvclass">)  [unwired: 6 in]
              }
              event "Go to Home": Value Change {
                n92 = event-data() -> ()  [unwired: 1 in, 6 out]
                n93 = call-dynamic "sendCommand.vi"("error in (no error)"=w317, "Command"="DPOS=0", "Axis Letter"=w318, "Controller in"=w319) -> ("error out"=w316:errorcluster, "Controller out"=w314:refnum<class "Controller.lvclass">)  [unwired: 6 in]
              }
              event "Scan Right": Value Change {
                n94 = event-data() -> ()  [unwired: 1 in, 6 out]
                n95 = call-dynamic "sendCommand.vi"("error in (no error)"=w323, "Command"="SCAN=1", "Axis Letter"=w324, "Controller in"=w325) -> ("error out"=w322:errorcluster, "Controller out"=w321:refnum<class "Controller.lvclass">)  [unwired: 6 in]
              }
              event "Scan Left": Value Change {
                n96 = event-data() -> ()  [unwired: 1 in, 6 out]
                n97 = call-dynamic "sendCommand.vi"("error in (no error)"=w329, "Command"="SCAN=-1", "Axis Letter"=w330, "Controller in"=w331) -> ("error out"=w328:errorcluster, "Controller out"=w327:refnum<class "Controller.lvclass">)  [unwired: 6 in]
              }
              event "Continue": Value Change {
                n98 = event-data() -> ()  [unwired: 1 in, 6 out]
                n99 = call-dynamic "sendCommand.vi"("error in (no error)"=w335, "Command"="CONT=0", "Axis Letter"=w336, "Controller in"=w337) -> ("error out"=w334:errorcluster, "Controller out"=w333:refnum<class "Controller.lvclass">)  [unwired: 6 in]
              }
              event "Stop": Value Change {
                n100 = event-data() -> ()  [unwired: 1 in, 6 out]
                n101 = call-dynamic "sendCommand.vi"("error in (no error)"=w341, "Command"="STOP=0", "Axis Letter"=w342, "Controller in"=w343) -> ("error out"=w340:errorcluster, "Controller out"=w339:refnum<class "Controller.lvclass">)  [unwired: 6 in]
              }
              event "Make Step Right": Value Change {
                n102 = event-data() -> ()  [unwired: 1 in, 6 out]
                n103 = call-dynamic "setStep.vi"("error in (no error)"=w348, "Step Value"=w349, "Axis Letter"=w346, "Controller in"=w347) -> ("error out"=w344:errorcluster, "Controller out"=w345:refnum<class "Controller.lvclass">)  [unwired: 6 in]
              }
              event "Step Size \n[selected units]": Value Change {
                n104 = event-data() -> ()  [unwired: 1 in, 6 out]
              }
              event "Make Step Left": Value Change {
                n105 = event-data() -> ()  [unwired: 1 in, 6 out]
                n106 = Multiply(x=-1, y=w358) -> (x*y=w355:dbl)
                n107 = call-dynamic "setStep.vi"("error in (no error)"=w354, "Step Value"=w355, "Axis Letter"=w356, "Controller in"=w357) -> ("error out"=w353:errorcluster, "Controller out"=w352:refnum<class "Controller.lvclass">)  [unwired: 6 in]
              }
              event "Desired Speed \n[1µm/s or 0,01deg /s]": Value Change {
                n108 = event-data() -> ()  [unwired: 1 in, 6 out]
                n109 = Number To Decimal String(number=w365) -> (decimal integer string=w363:string)  [unwired: 1 in]
                n110 = Concatenate Strings("SSPD=", w363) -> (w362:string)
                n111 = call-dynamic "sendCommand.vi"("error in (no error)"=w366, "Command"=w362, "Axis Letter"=w367, "Controller in"=w368) -> ("error out"=w361:errorcluster, "Controller out"=w360:refnum<class "Controller.lvclass">)  [unwired: 6 in]
              }
              event "Find Index": Value Change {
                n112 = event-data() -> ()  [unwired: 1 in, 6 out]
                n113 = call-dynamic "sendCommand.vi"("error in (no error)"=w372, "Command"="INDX=0", "Axis Letter"=w373, "Controller in"=w374) -> ("error out"=w371:errorcluster, "Controller out"=w370:refnum<class "Controller.lvclass">)  [unwired: 6 in]
              }
              event "Reset": Value Change {
                n114 = event-data() -> ()  [unwired: 1 in, 6 out]
                n115 = call-dynamic "sendCommand.vi"("error in (no error)"=w379, "Command"="RSET=0", "Axis Letter"=w378, "Controller in"=w380) -> ("error out"=w375:errorcluster, "Controller out"=w376:refnum<class "Controller.lvclass">)  [unwired: 6 in]
              }
              event "Axis Resolution 2": Value Change {
                n116 = event-data() -> ()  [unwired: 1 in, 6 out]
              }
            }
          }
          frame "Settings" {
          }
        }
        n117 = node-c288() -> ()  [unwired: 1 in, 1 out]
      }
      n118 = node-c288(w55) -> ()  [unwired: 1 out]
      n119 = Merge Errors(w54, w52) -> (w53:errorcluster)
    }
  }
  "error out" <- w11
